vi "Calculate_ramp_rate.vi"(4 "Phi (Deg)":dbl format="%#_13g", 5 "H_final (T)":dbl format="%#_13g", 6 "Phi_init (Deg)":dbl format="%#_13g", 7 "H_init (T)":dbl format="%#_13g") -> (0 "Z-Ramp":dbl format="%#_13g", 1 "Y-Ramp":dbl format="%#_13g")   [LabVIEW 2019]
uses:
  Global/Global Variables/global.vi
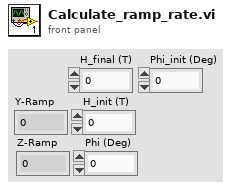
[diagram p1: front panel]
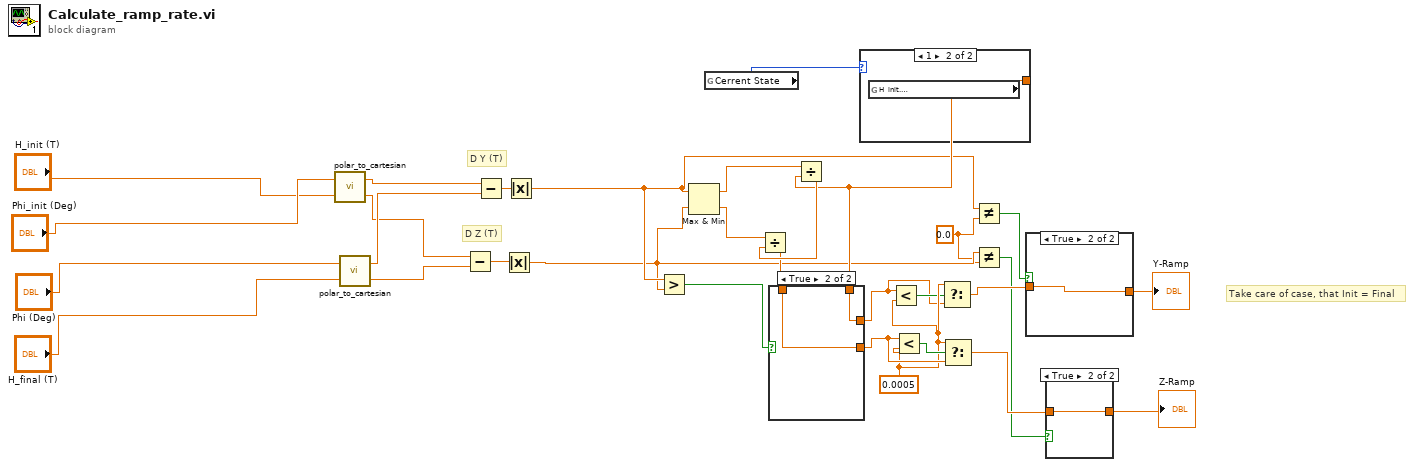
[diagram p0: block diagram]
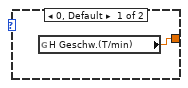
[diagram p2: hidden frame]
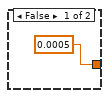
[diagram p3: hidden frame]
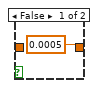
[diagram p4: hidden frame]
diagram:
  w6 = 0.0
  w16 = 0.0005
  # "Take care of case, that Init = Final"
  # "D Z (T)"
  # "D Y (T)"
  n1 = call "polar_to_cartesian.vi"("B (T)"="H_init (T)", "Phi (Deg)"="Phi_init (Deg)") -> ("Z Field (T)"=w29:dbl, "Y Field (T)"=w31:dbl)
  n2 = call "polar_to_cartesian.vi"("B (T)"="H_final (T)", "Phi (Deg)"="Phi (Deg)") -> ("Z Field (T)"=w28:dbl, "Y Field (T)"=w30:dbl)
  n3 = Subtract(x=w29, y=w28) -> (x-y=w20:dbl)
  n4 = Subtract(x=w31, y=w30) -> (x-y=w21:dbl)
  n5 = Absolute Value(x=w20) -> (abs(x)=w7:dbl)
  n6 = Absolute Value(x=w21) -> (abs(x)=w8:dbl)
  n7 = Greater?(x=w8, y=w7) -> (0:w24:bool)
  n8 = Max & Min(x=w8, y=w7) -> (max(x,y)=w27:dbl, min(x,y)=w26:dbl)
  n9 = global read "global.vi" "Cerrent State"() -> (w1:i32)
  n10 = case shown="1" w1 {
    tunnel: [w32 w33] -> w23
    frame 0, Default {
      n11 = global read "global.vi" "H Geschw.(T/min)"() -> (w32:dbl)
    }
    frame 1 {
      n12 = global read "global.vi" "H  init. \nGeschw.(T/min)"() -> (w33:dbl)
    }
  }
  n13 = Divide(x=w27, y=w23) -> (x/y=w25:dbl)
  n14 = Divide(x=w26, y=w25) -> (x/y=w22:dbl)
  n15 = case shown="True" w24 {
    tunnel: [w34 w37] -> w14
    tunnel: w23 -> [w35 w37]
    tunnel: w22 -> [w34 w36]
    tunnel: [w35 w36] -> w18
    frame False {
    }
    frame True {
    }
  }
  n16 = Less?(x=w14, y=w16) -> (x < y?=w15:bool)
  n17 = Less?(x=w18, y=w16) -> (x < y?=w17:bool)
  n18 = Select(t=w16, s=w15, f=w14) -> (s? t:f=w13:dbl)
  n19 = Select(t=w16, s=w17, f=w18) -> (s? t:f=w19:dbl)
  n20 = Not Equal?(x=w8, y=w6) -> (x != y?=w5:bool)
  n21 = Not Equal?(x=w7, y=w6) -> (x != y?=w4:bool)
  n22 = case shown="True" w5 {
    tunnel: w13 -> [_ w39]
    tunnel: [0.0005 w39] -> w3
    frame False {
    }
    frame True {
    }
  }
  "Y-Ramp" <- w3
  n23 = case shown="True" w4 {
    tunnel: w19 -> [_ w41]
    tunnel: [0.0005 w41] -> w2
    frame False {
    }
    frame True {
    }
  }
  "Z-Ramp" <- w2
